vi "ConfigureController.vi"(8 "error in (no error)":errorcluster, 11 "VISA resource name":refnum<visa-resource-name>) -> (0 "error out":errorcluster, 3 "VISA resource name out":refnum<visa-resource-name>)   [LabVIEW 2018]
uses:
  <vilib>/Instr/_visa.llb/VISA Configure Serial Port (Instr).vi
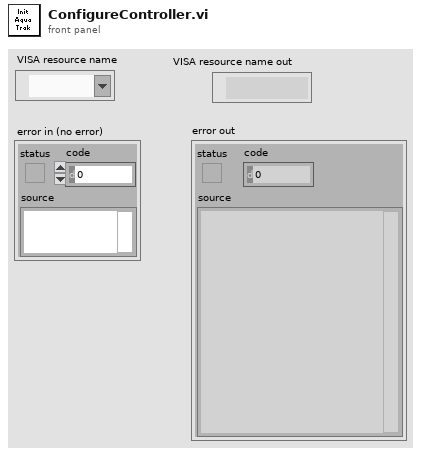
[diagram p1: front panel]
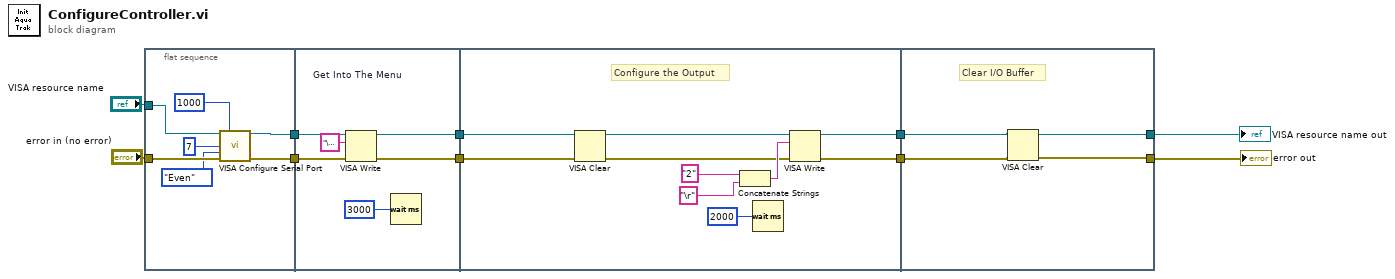
[diagram p0: block diagram]
diagram:
  n1 = flat-sequence {
    tunnel: "error in (no error)" -> [w15]
    tunnel: "VISA resource name" -> [w17]
    tunnel: [w16] -> w2
    tunnel: [w14] -> w1
    tunnel: [w20] -> w10
    tunnel: [w19] -> w9
    tunnel: w2 -> [w22]
    tunnel: w1 -> [w21]
    tunnel: w10 -> [w28]
    tunnel: w9 -> [w27]
    tunnel: [w31] -> w8
    tunnel: [w30] -> w7
    tunnel: [w35] -> w5
    tunnel: [w34] -> w6
    tunnel: w8 -> [w36]
    tunnel: w7 -> [w37]
    frame #0 {
      n2 = call-poly "VISA Configure Serial Port"("VISA resource name"=w17, "timeout (10sec)"=u32 1000, "data bits (8)"=u16 7, "parity (0:none)"=enum16{"None", "Odd", "Even", "Mark", "Space"}."Even", "error in (no error)"=w15) -> ("VISA resource name out"=w16:refnum<visa-resource-name>, "error out"=w14:errorcluster)  [unwired: 9 in]
    }
    frame #1 {
      w23 = "\u001b"  # Get Into The Menu
      n3 = VISA Write(VISA resource name=w22, write buffer=w23, error in (no error)=w21) -> (VISA resource name out=w20:refnum<visa-resource-name>, error out=w19:errorcluster)  [unwired: 1 out]
      n4 = Wait (ms)(milliseconds to wait=u32 3000 ("millisecond multiple")) -> ()  [unwired: 1 out]
    }
    frame #2 {
      # "Configure the Output"
      n5 = VISA Clear(VISA resource name=w28, error in (no error)=w27) -> (VISA resource name out=w26:refnum<visa-resource-name>, error out=w25:errorcluster)
      n6 = Concatenate Strings("2" ("string"), "\r") -> (w32:string)
      n7 = Wait (ms)(milliseconds to wait=u32 2000 ("millisecond multiple")) -> ()  [unwired: 1 out]
      n8 = VISA Write(VISA resource name=w26, write buffer=w32, error in (no error)=w25) -> (VISA resource name out=w30:refnum<visa-resource-name>, error out=w31:errorcluster)  [unwired: 1 out]
    }
    frame #3 {
      # "Clear I/O Buffer"
      n9 = VISA Clear(VISA resource name=w37, error in (no error)=w36) -> (VISA resource name out=w35:refnum<visa-resource-name>, error out=w34:errorcluster)
    }
  }
  "error out" <- w6
  "VISA resource name out" <- w5
